vi "From Binary.vi"(6 "byte order":T1(ring), 8 "error in (no error)":errorcluster, 10 "Binary":string, 11 "Double Float in":refnum<class "Abs_Complex Extended Float.lvclass">) -> (0 "error out":errorcluster, 2 "Remaining":string, 3 "Double Float out":refnum<class "Abs_Complex Extended Float.lvclass">)   [LabVIEW 2021, in "Abs_Complex Extended Float.lvclass"]
uses:
  Abs_Complex Extended Float.lvclass
  Support/Type.ctl
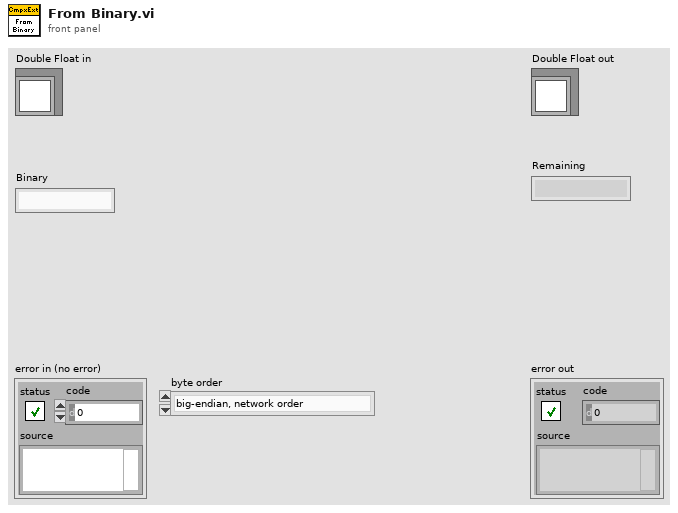
[diagram p1: front panel]
types:
  T1 = enum16{"big-endian, network order", "native, host order", "little-endian"}
  T2 = typedef "Abs_Complex Extended Float.lvclass/Type.ctl" = cxt
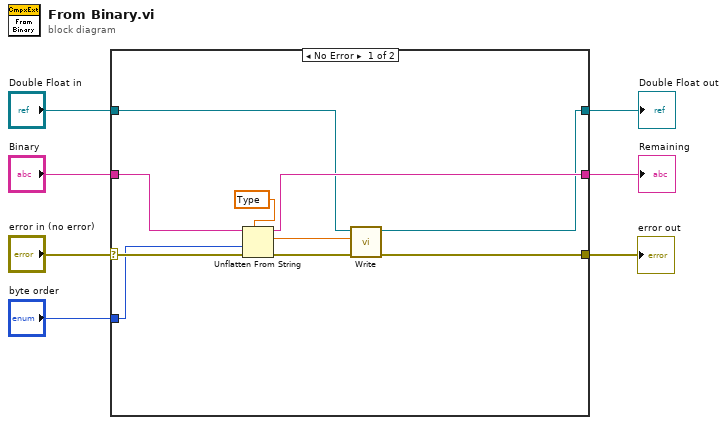
[diagram p0: block diagram]
diagram:
  n1 = case shown="No Error" "error in (no error)" {
    selector: "error in (no error)" -> [w15 w19]
    tunnel: [w11 w19] -> w2
    tunnel: [w9 w20] -> w3
    tunnel: "byte order" -> [w14 _]
    tunnel: "Double Float in" -> [w10 w20]
    tunnel: "Binary" -> [w17 w18]
    tunnel: [w16 w18] -> w1
    frame No Error {
      n2 = Unflatten From String(type=T2 0.0+0.0i, binary string=w17, byte order (0:big-endian, network order)=w14, error in (no error)=w15) -> (rest of the binary string=w16:string, value=w13:T2, error out=w12:errorcluster)  [unwired: 1 in]
      n3 = call-dynamic "Write.vi"("error in (no error)"=w12, "Value"=w13, "Double Float.lvclass_340760 in"=w10) -> ("error out"=w11:errorcluster, "Double Float.lvclass_340760 out"=w9:refnum<class "Abs_Complex Extended Float.lvclass">)  [unwired: 7 in]
    }
    frame Error {
    }
  }
  "error out" <- w2
  "Double Float out" <- w3
  "Remaining" <- w1
